vi "ini_sesion.vi"(8 "error in (no error)":errorcluster, 11 "USRP_1_x_200MHz in":refnum<class "USRP_1_x_200MHz.lvclass">) -> (0 "error out":errorcluster, 3 "USRP_1_x_200MHz out":refnum<class "USRP_1_x_200MHz.lvclass">)   [LabVIEW 2021, in "USRP_1_x_200MHz.lvclass"]
uses:
  USRP_1_x_200MHz.lvclass
  <instrlib>/niUsrpRio/Config/v1/Host/Private/LO Source.ctl
  USRP_1_x_200MHz.lvclass/USRP_1_x_200MHz.ctl
  <vilib>/FPGAPlugInAG/USRP 294xR; 295xR 200 MSps/niLvFpga_Open_USRP 294xR; 295xR 200 MSps.vi
  <vilib>/rvi/interface/common/dynamic/niFpgaDynamicAddResources.vi
  <vilib>/Utility/error.llb/Error Cluster From Error Code.vi
  <vilib>/rvi/errors/niLvFpgaAdjustHostInterfaceError.vi
  <vilib>/rvi/interface/common/niFpgaWaitOnOcc.vi
  <vilib>/rvi/interface/nirviOpenFPGA/nirviOpenFPGA.xnode
  FPGA Bitfiles/USRP_Multi_Emitter_one_channel.lvbitx
  <vilib>/rvi/interface/nirviReadWriteControl/nirviReadWriteControl.xnode
  <vilib>/rvi/interface/nirviMethod/nirviMethod.xnode
  <vilib>/FPGAPlugInAG/Dynamic/niLvFpga_ConfigureFifo_Dynamic.vi
  <vilib>/rvi/errors/niLvFpgaMergeErrorWithErrorCode.vi
  NiFpgaLv.dll
  <vilib>/rvi/interface/Simulation/niFpgaSimulationCallBeginRW.vi
  <instrlib>/niUsrpRio/Config/v1/Host/niUsrpRio Config v1 Host.lvlib
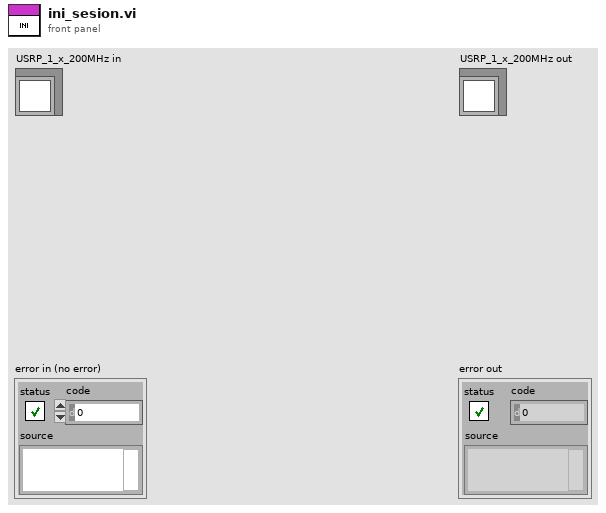
[diagram p1: front panel]
types:
  T1 = cluster{"gain I":fxp<+/-,24,3>, "gain Q":fxp<+/-,24,3>}
  T2 = typedef "niUsrpRio Config v1 Host.lvlib/LO Source.ctl" = enum16{"Internal", "Companion", "External", "Reimport"}
  T3 = typedef "nirio_resource_hc.ctl" = tag
  T4 = typedef "niUsrpRio Config v1 Host.lvlib/niUsrpRio Session.ctl" = cluster{"FPGA Interface":refnum<k20>, "RIO Interface Number":u32, "Data Clock Rate":u32, "FPGA Data Clock Rate":u32, "Global Settings Register Bus":T5, "Radio 0 Settings Register Bus":T5, "Radio 1 Settings Register Bus":T5, "Radio Settings Bus Semaphore":T6, "DB Queues":T7[], "Characterization Data Valid?":bool, "EEPROM Header":T8, "Device Data Header":T9, "EEPROM Characterization Header":T10, "Characterization Data":T11[], "FPGA Current Version":u32, "FPGA Oldest Compatible Version":u32, "Fixed Logic Current Version":u32, "Fixed Logic Oldest Compatible Version":u32, "FPGA Radio Settings Bus Current Version":u32, "FPGA Radio Settings Bus Oldest Compatible Version":u32, "FPGA Board Config Current Version":u32, "FPGA Board Config Oldest Compatible Version":u32, "Daughterboard Clock Rate":u32, "daughterboard configuration session handles":u64[]}
  T5 = typedef "niInstr Register Bus v0 Host.lvlib/Register Bus Session.ctl" = refnum<queue>
  T6 = typedef "Semaphore RefNum" = refnum<k1>
  T7 = typedef "niUsrpRio Config v1 Host.lvlib/DB Queue Reference.ctl" = refnum<queue>
  T8 = typedef "niUsrpRio Config v1 Host.lvlib/EEPROM Header.ctl" = cluster{"Checksum":u32, "Product Code":u16, "Hardware Current Version":u16, "Hardware Oldest Compatible Version":u16, "EEPROM Map Current Version":u16, "EEPROM Map Oldest Compatible Version":u16, "User Password":string, "Pointer to Factory Header":u32, "Pointer to User Header":u32, "Recommended Interval":u16, "Number of Reserved Bytes":i32, "Number of Daughterboards":u8, "Daughterboard IDs":u16[], "Daughterboard Serial Numbers":string[]}
  T9 = typedef "niUsrpRio Config v1 Host.lvlib/EEPROM Device Data Header.ctl" = cluster{"Checksum":u32, "Number of Channels":u8, "Number of Gain Settings":u16[], "Pointer to Characterization Data":u32[], "Number of Reserved Bytes":i32, "Number of Frequencies":u16[]}
  T10 = typedef "niUsrpRio Config v1 Host.lvlib/EEPROM Characterization Header.ctl" = cluster{"Checksum":u32, "Date":timestamp, "Temperature":sgl, "Misc. Info":string, "Pointer to Device Data Header":u32, "Number of Reserved Bytes":i32}
  T11 = typedef "niUsrpRio Config v1 Host.lvlib/Characterization Data.ctl" = cluster{"Gains[dB]":dbl[], "Frequencies [Hz]":dbl[], "IQ Imbalance Table":T12[], "Measured Gains[dB]":dbl[][]}
  T12 = typedef "niUsrpRio Config v1 Host.lvlib/IQ Imbalance.ctl" = cluster{"Gain Imbalance [linear]":dbl, "Phase Imbalance [radians]":dbl, "Offset":cdb}
  T13 = typedef "niInstr DSP v1 Shared.lvlib/IQ Impairments.ctl" = cluster{"inline gain I":fxp<+/-,18,1>, "inline gain Q":fxp<+/-,18,1>, "cross gain I":fxp<+/-,18,1>, "cross gain Q":fxp<+/-,18,1>, "pre-gain offset I":fxp<+/-,18,1>, "pre-gain offset Q":fxp<+/-,18,1>, "post-gain offset I":fxp<+/-,18,1>, "post-gain offset Q":fxp<+/-,18,1>}
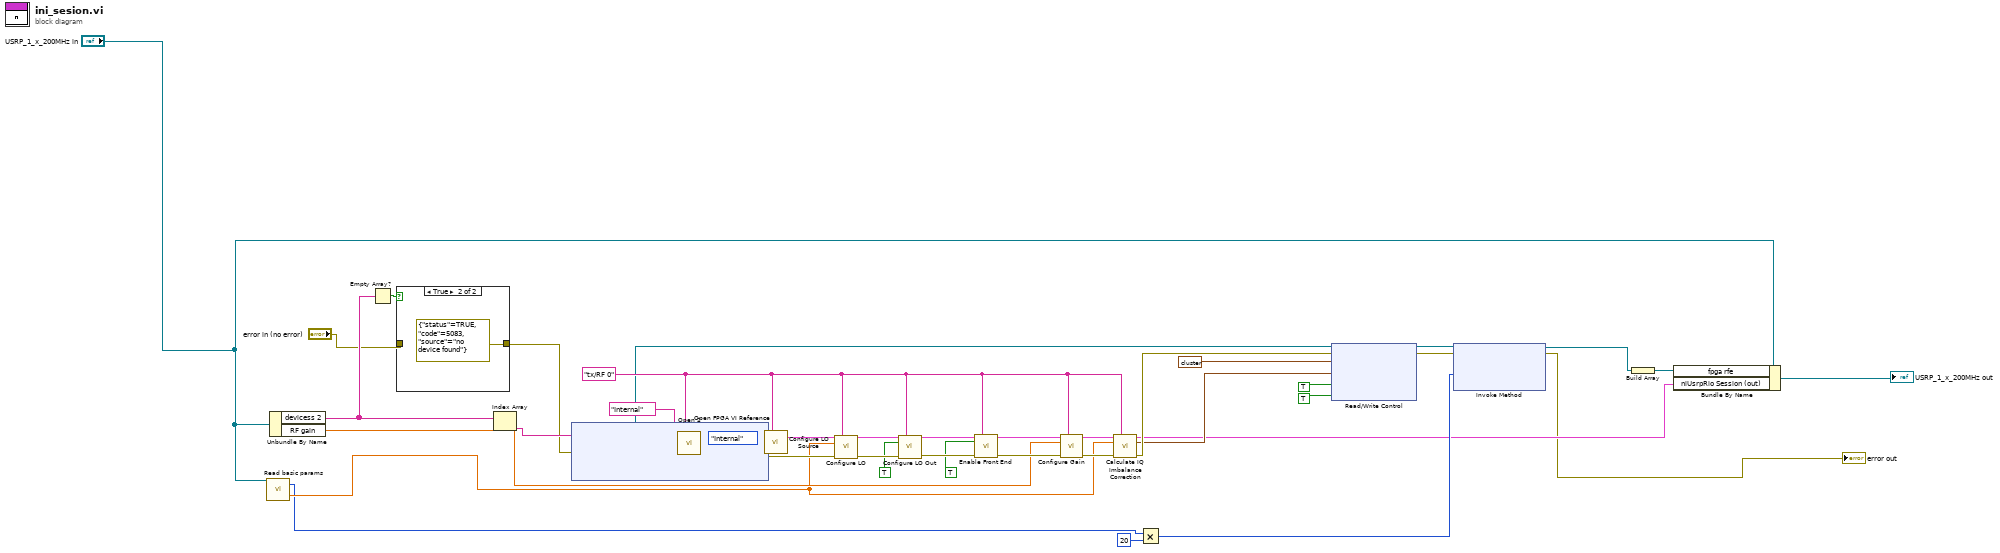
[diagram p0: block diagram]
diagram:
  w17 = "tx/RF 0" ("scope")
  n1 = call-dynamic "Read basic params.vi"("device_type in"="USRP_1_x_200MHz in") -> ("buffer size"=w3:u32, "center frequency (Hz)"=w4:dbl)  [unwired: 13 in, 4 out]
  n2 = Unbundle By Name("USRP_1_x_200MHz in") -> ("devicess 2"=w8:T3[], "RF gain"=w10:dbl)
  n3 = Empty Array?(array=w8) -> (empty?=w9:bool)
  n4 = case shown="True" w9 {
    tunnel: [w43 errorcluster {"status"=TRUE, "code"=5083, "source"="no device found"} ("error in (no error)")] -> w7
    tunnel: "error in (no error)" -> [w43 _]
    frame False {
    }
    frame True {
    }
  }
  n5 = Index Array(array=w8) -> (element=w37:T3)  [unwired: 1 in]
  n6 = xnode ("Open FPGA VI Reference")("error in"=w7, "resource name"=w37) -> ("FPGA VI Reference Out"=w16:refnum<k20>, "error out"=w38:errorcluster)
  n7 = call <instrlib>:"Open 2.vi"("fpga ref"=w16, "scope"=w17, "Reference Frequency Source"="Internal", "error in"=w38) -> ("niUsrpRio Session (out)"=w39:T4, "error out"=w41:errorcluster)  [unwired: 10 in]
  n8 = call <instrlib>:"Configure LO Source.vi"("niUsrpRio Session"=w39, "scope"=w17, "lo source"=LO_Source."Internal", "error in"=w41) -> ("niUsrpRio Session (out)"=w19:T4, "error out"=w18:errorcluster)  [unwired: 10 in]
  n9 = call <instrlib>:"Configure LO.vi"("niUsrpRio Session"=w19, "scope"=w17, "frequency"=w4, "error in"=w18) -> ("niUsrpRio Session (out)"=w36:T4, "error out"=w35:errorcluster)  [unwired: 8 in, 2 out]
  n10 = call <instrlib>:"Configure LO Out.vi"("niUsrpRio Session"=w36, "scope"=w17, "enable"=TRUE ("enable 0"), "error in"=w35) -> ("niUsrpRio Session (out)"=w33:T4, "error out"=w30:errorcluster)  [unwired: 10 in]
  n11 = call <instrlib>:"Enable Front End.vi"("niUsrpRio Session"=w33, "scope"=w17, "enable"=TRUE ("enable 0 2"), "error in"=w30) -> ("niUsrpRio Session (out)"=w32:T4, "error out"=w31:errorcluster)  [unwired: 10 in]
  n12 = call <instrlib>:"Configure Gain.vi"("niUsrpRio Session"=w32, "scope"=w17, "gain"=w10, "error in"=w31) -> ("niUsrpRio Session (out)"=w28:T4, "error out"=w27:errorcluster)  [unwired: 9 in, 1 out]
  n13 = call <instrlib>:"Calculate IQ Imbalance Correction.vi"("niUsrpRio Session"=w28, "scope"=w17, "frequency"=w4, "error in"=w27) -> ("niUsrpRio Session (out)"=w11:T4, "IQ imbalance correction"=w23:T13, "error out"=w26:errorcluster)  [unwired: 8 in, 1 out]
  n14 = Multiply(x=w3, y=u32 20) -> (x*y=w13:u32)
  n15 = xnode ("Read/Write Control")("FPGA VI Reference In"=w16, "error in"=w26, "tx.gain.0"=T1 {"gain I"=1.0, "gain Q"=1.0}, "tx.impairments.0"=w23, "reset system clock"=TRUE, "RF 0/Tx/Enable"=TRUE) -> ("FPGA VI Reference Out"=w21:refnum<k20>, "error out"=w20:errorcluster)
  n16 = xnode ("Invoke Method")("FPGA VI Reference In"=w21, "error in"=w20, "Requested Depth"=w13) -> ("FPGA VI Reference Out"=w15:refnum<k20>, "error out"=→"error out":errorcluster)  [unwired: 1 out]
  n17 = Build Array(w15) -> (w12:refnum<k20>[])
  n18 = Bundle By Name(cluster="USRP_1_x_200MHz in", "fpga rfe"=w12, "niUsrpRio Session (out)"=w11) -> (→"USRP_1_x_200MHz out":refnum<class "USRP_1_x_200MHz.lvclass">)
